vi "A170316-11_Auto.vi"() -> ()   [LabVIEW 2020]
uses:
  Global_Variable/A170316-11.vi
  Global_Variable/Global.vi
  Database/Global1.vi
  <vilib>/addons/database/Connection.llb/DB Tools Open Connec (String).vi
  <vilib>/addons/database/NI_Database_API.lvlib
panel:
  in  "前序OK？":string
  out "拾取检具14":bool
  out "拾取检具13":bool
  out "拾取检具12":bool
  out "拾取检具11":bool
  out "拾取检具10":bool
  out "拾取检具9":bool
  out "拾取检具8":bool
  out "拾取检具7":bool
  out "拾取检具6":bool
  out "拾取检具5":bool
  out "拾取检具4":bool
  out "拾取检具3":bool
  out "拾取检具2":bool
  out "拾取检具1":bool
  out "磨合次数":i32
  in  "STEP":string
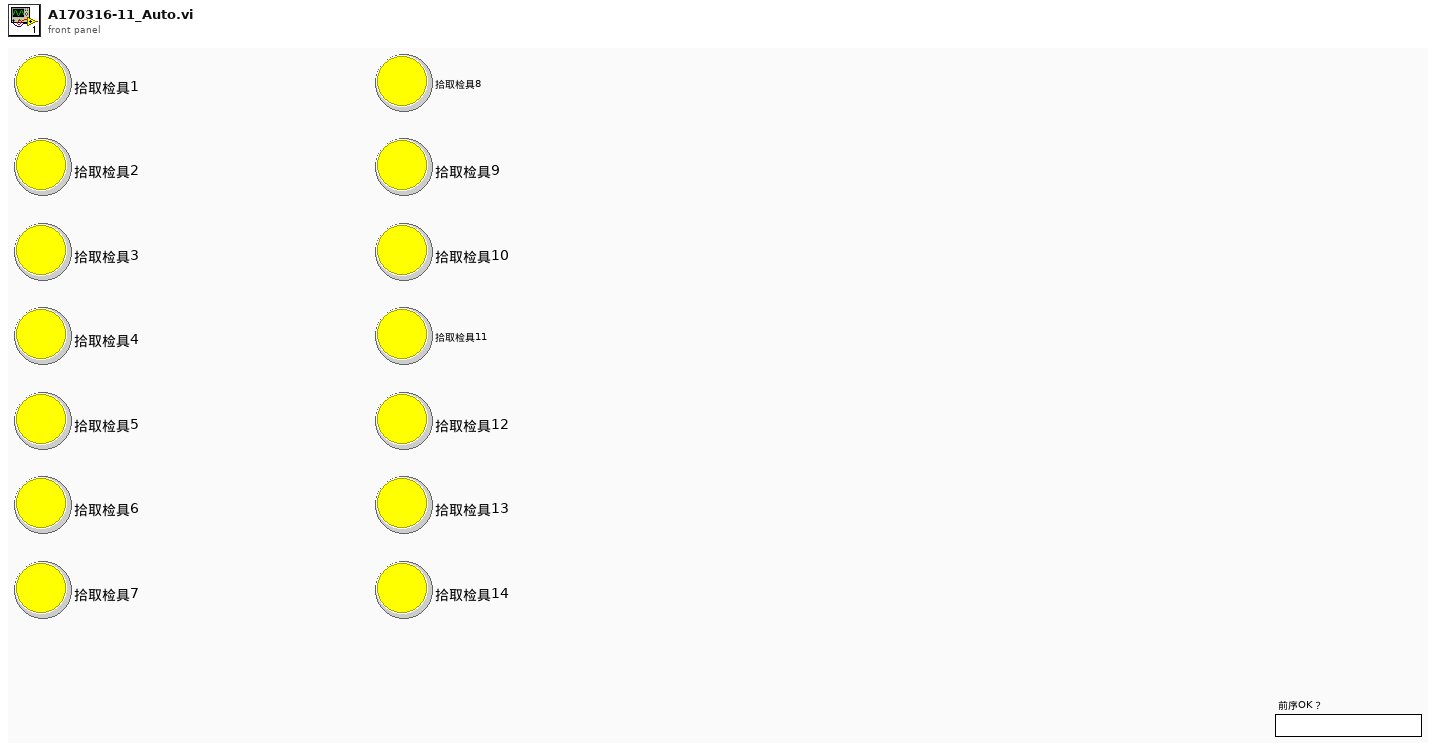
[diagram p1: front panel]
types:
  T1 = enum32{"Invalid", "Standard", "Closed", "Hidden", "Minimized", "Maximized"}
  T2 = cluster{i64, i64, i64, "生产结果":string, "result string":string}
  T3 = cluster{i64, i64, i64, "生产结果":string, "result string":string}[]
  T4 = typedef "NI_Database_API.lvlib/Conn ObjectReference.ctl" = refnum<k1>
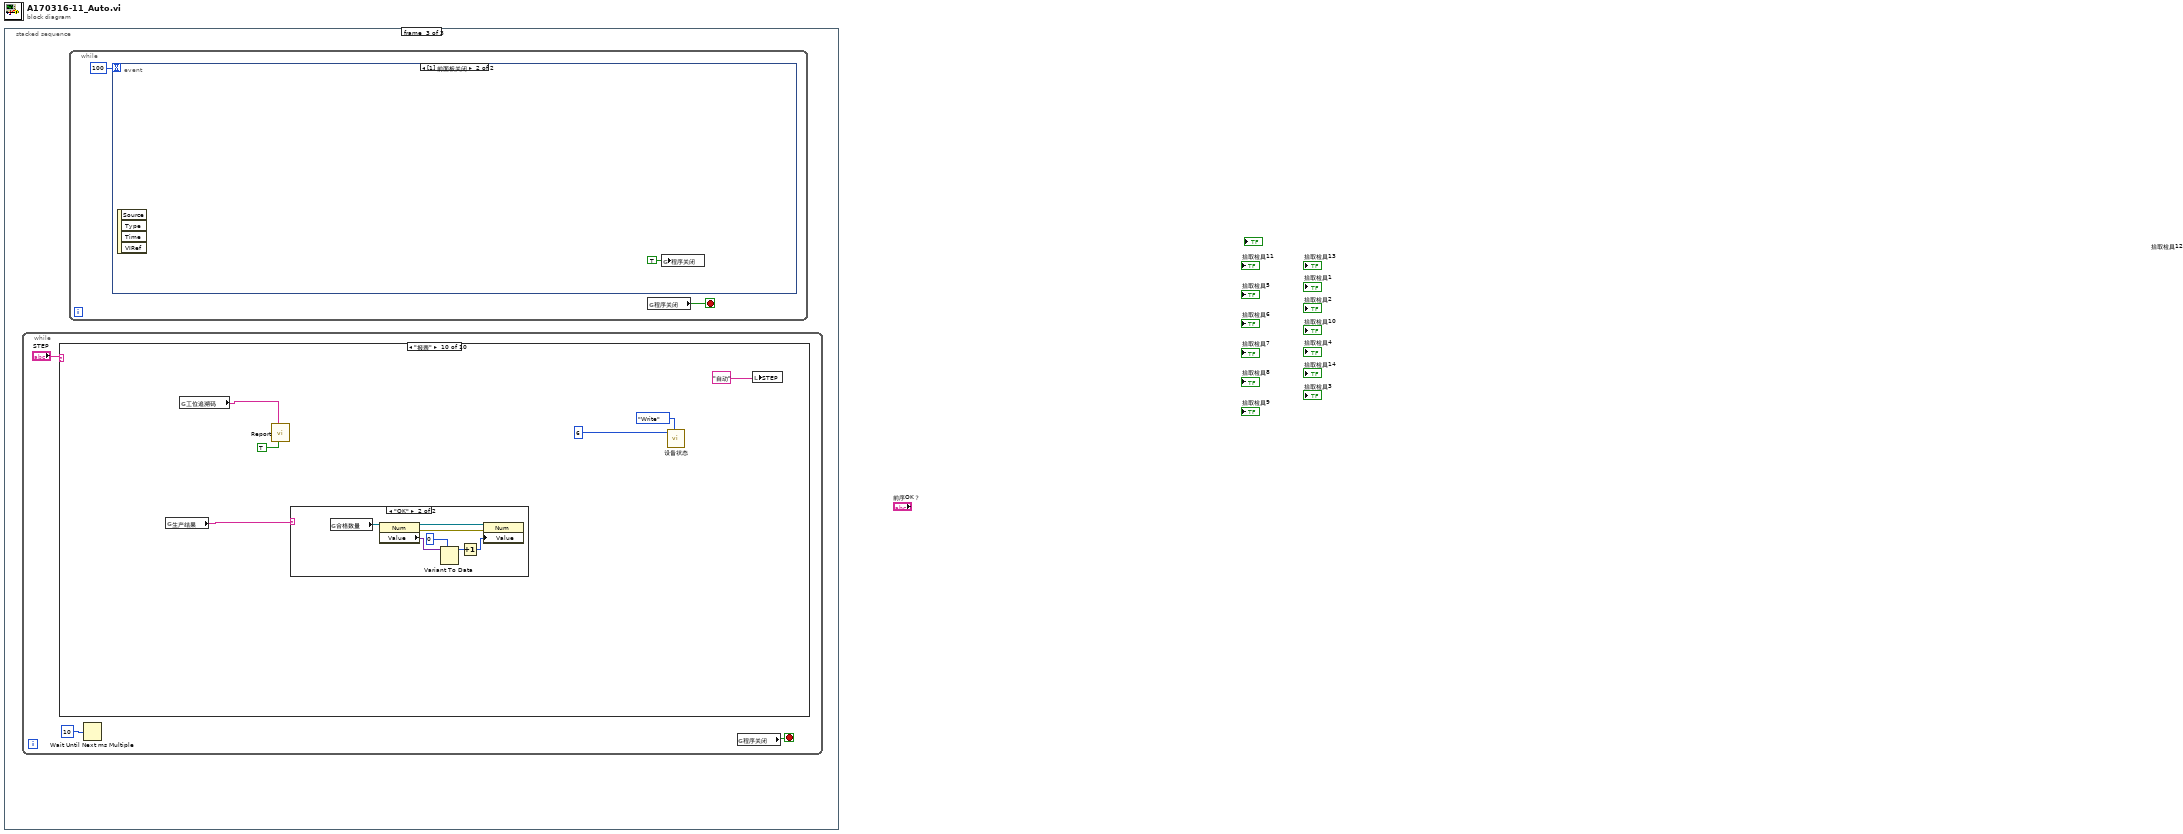
[diagram p0: block diagram]
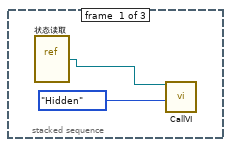
[diagram p2: hidden frame]
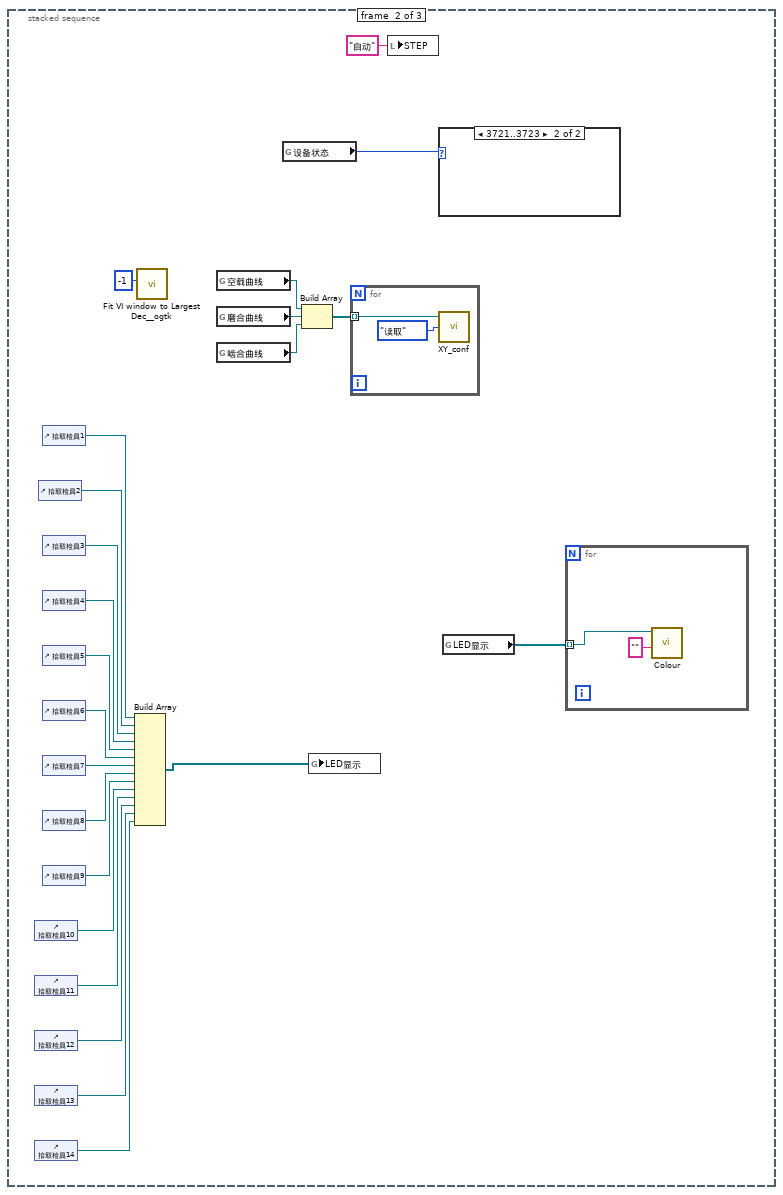
[diagram p3: hidden frame]
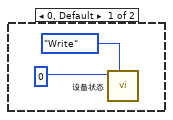
[diagram p4: hidden frame]
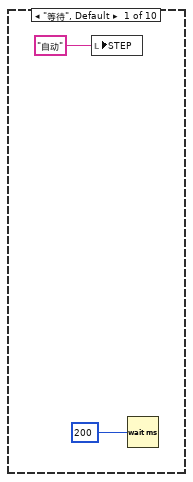
[diagram p5: hidden frame]
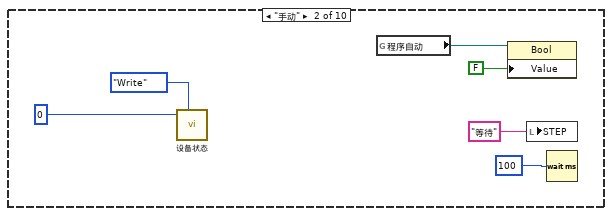
[diagram p6: hidden frame]
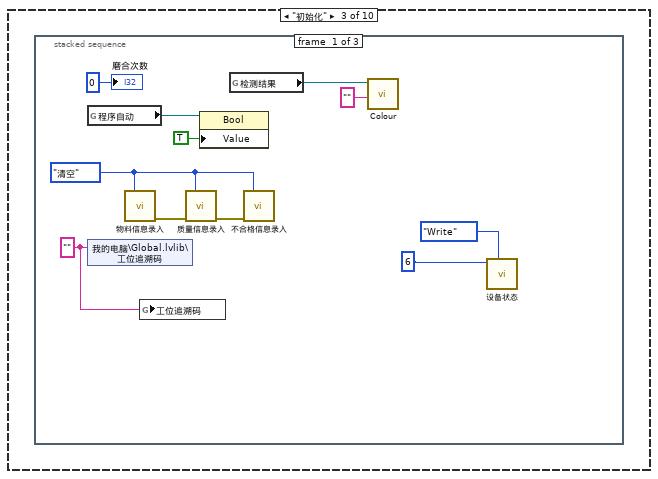
[diagram p7: hidden frame]
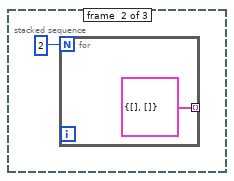
[diagram p8: hidden frame]
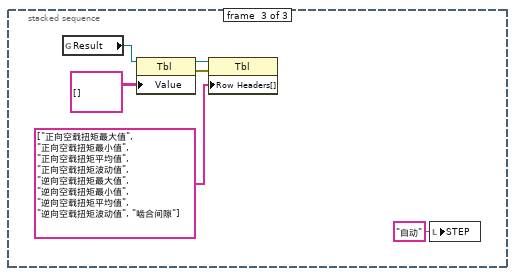
[diagram p9: hidden frame]
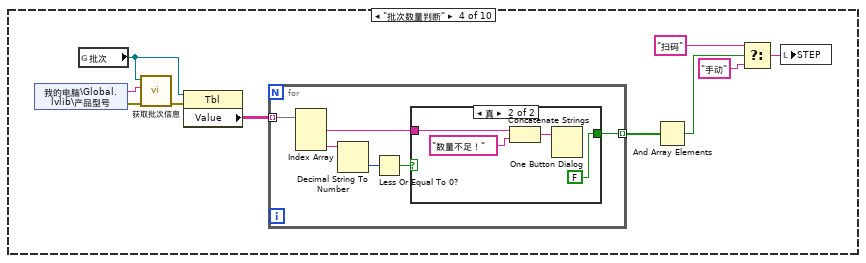
[diagram p10: hidden frame]
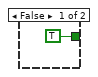
[diagram p11: hidden frame]
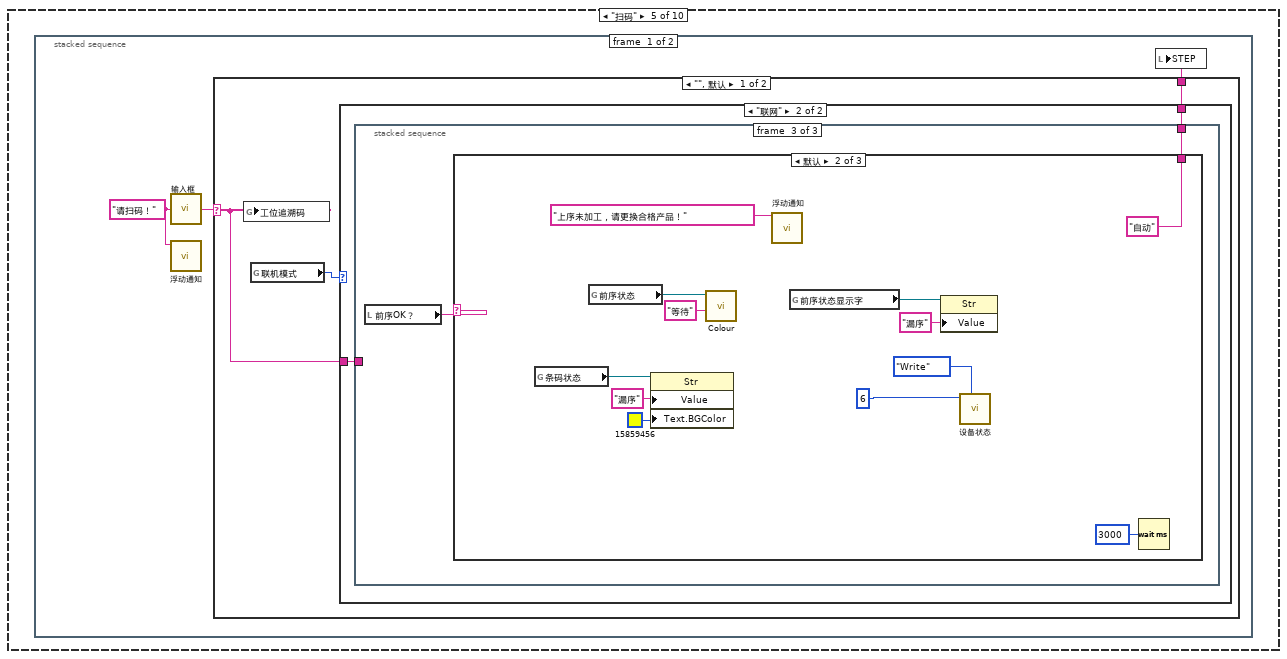
[diagram p12: hidden frame]
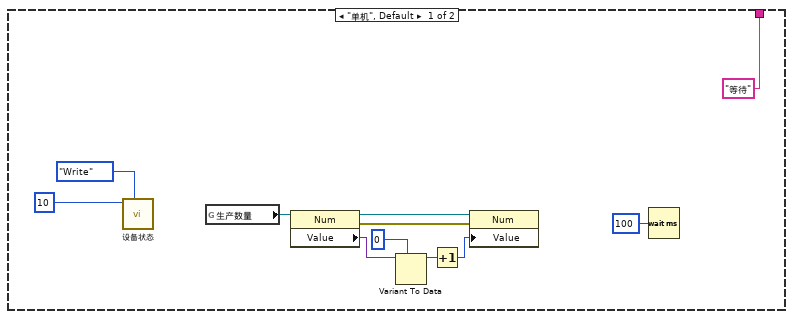
[diagram p13: hidden frame]
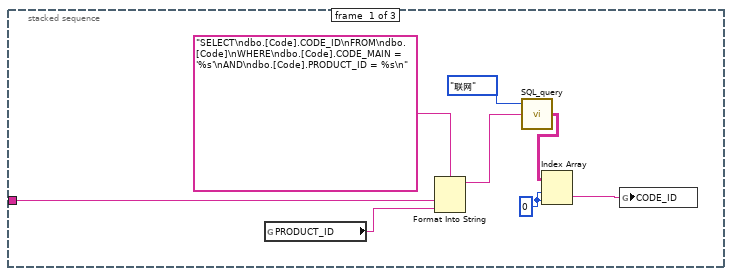
[diagram p14: hidden frame]
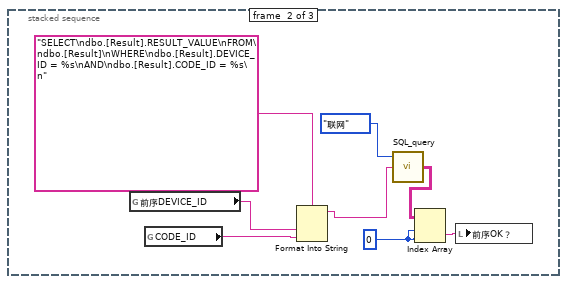
[diagram p15: hidden frame]
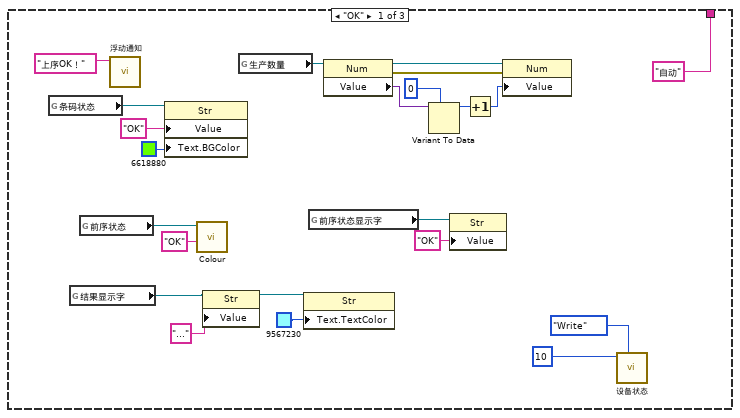
[diagram p16: hidden frame]
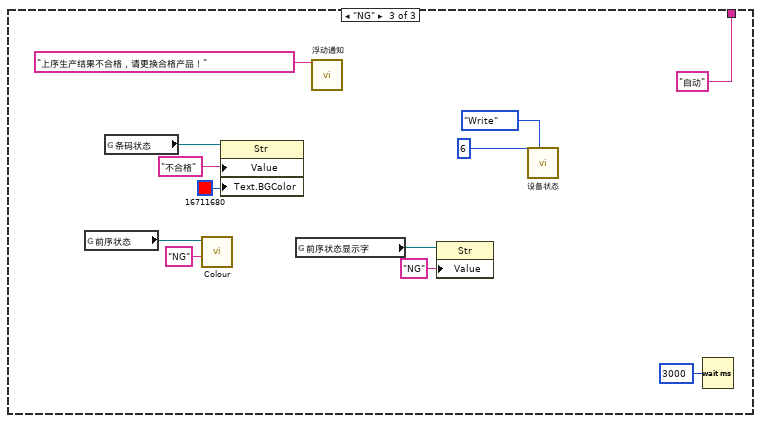
[diagram p17: hidden frame]
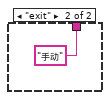
[diagram p18: hidden frame]
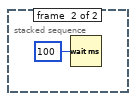
[diagram p19: hidden frame]
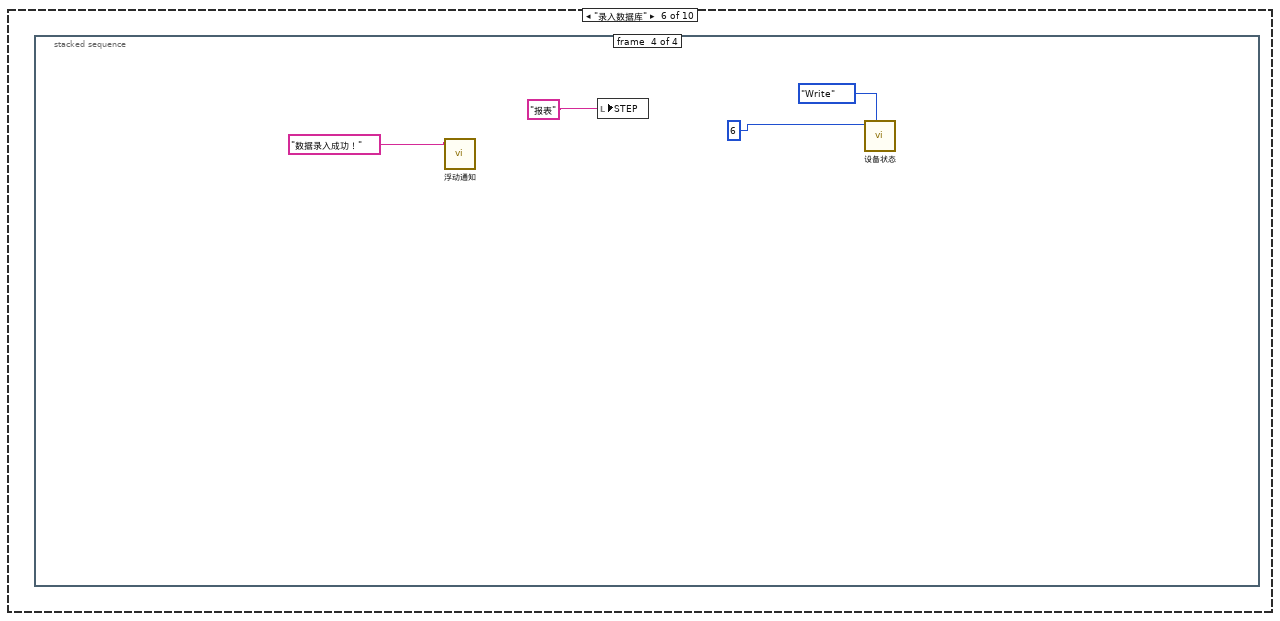
[diagram p20: hidden frame]
diagram:
  n1 = stacked-sequence {
    frame #0 {
      n2 = vi-ref "状态读取.vi"() -> (w1:refnum<vi>)
      n3 = call "CallVI.vi"("VI引用"=w1, "状态"=T1."Hidden") -> ()  [unwired: 11 in, 3 out]
    }
    frame #1 {
      n4 = control-ref of="拾取检具10"() -> (w10:refnum<vi>)
      n5 = control-ref of="拾取检具11"() -> (w9:refnum<vi>)
      n6 = control-ref of="拾取检具12"() -> (w8:refnum<vi>)
      n7 = control-ref of="拾取检具13"() -> (w7:refnum<vi>)
      n8 = control-ref of="拾取检具14"() -> (w6:refnum<vi>)
      n9 = control-ref of="拾取检具2"() -> (w18:refnum<vi>)
      n10 = control-ref of="拾取检具1"() -> (w19:refnum<vi>)
      n11 = control-ref of="拾取检具3"() -> (w17:refnum<vi>)
      n12 = control-ref of="拾取检具4"() -> (w16:refnum<vi>)
      n13 = control-ref of="拾取检具5"() -> (w15:refnum<vi>)
      n14 = control-ref of="拾取检具6"() -> (w14:refnum<vi>)
      n15 = control-ref of="拾取检具7"() -> (w13:refnum<vi>)
      n16 = control-ref of="拾取检具8"() -> (w12:refnum<vi>)
      n17 = control-ref of="拾取检具9"() -> (w11:refnum<vi>)
      n18 = Build Array(w19, w18, w17, w16, w15, w14, w13, w12, w11, w10, w9, w8, w7, w6) -> (w5:refnum<vi>[])
      n19 = call <userlib>:"Fit VI window to Largest Dec__ogtk.vi"("border spacing (2 px)"=-1) -> ()  [unwired: 5 in, 2 out]
      n20 = global read "A170316-11.vi" "空载曲线"() -> (w20:refnum<vi>)
      n21 = global read "A170316-11.vi" "磨合曲线"() -> (w21:refnum<vi>)
      n22 = global read "A170316-11.vi" "啮合曲线"() -> (w22:refnum<vi>)
      n23 = global read "Global.vi" "设备状态"() -> (w3:i32)
      n24 = Build Array(w20, w21, w22) -> (w24:refnum<vi>[])
      n25 = global write "A170316-11.vi" "LED显示"(w5) -> ()
      n26 = for {
        tunnel: w24 -> [w31] mode=indexing
        n27 = call "XY_conf.vi"("方式"=enum16{"写入", "读取"}."读取", "XY图引用"=w31) -> ()  [unwired: 3 in, 1 out]
      }
      n28 = local write "STEP"("自动" ("STEP")) -> ()
      n29 = case shown="3721..3723" w3 {
        frame 0, Default {
          n30 = call "设备状态.vi"("枚举"=enum16{"Read", "Write"}."Write", "Status_Write"=i16 0 ("设备状态")) -> ()  [unwired: 9 in, 1 out]
        }
        frame 3721..3723 {
        }
      }
      n31 = global read "A170316-11.vi" "LED显示"() -> (w4:refnum<vi>[])
      n32 = for {
        tunnel: w4 -> [w27] mode=indexing
        n33 = call "Colour.vi"("result"="", "colourRef"=w27) -> ()  [unwired: 9 in, 1 out]
      }
    }
    frame #2 {
      n34 = while {
        stop <- w33 stop-if-true
        n35 = case shown="\"报表\"" "STEP" {
          frame "等待", Default {
            n36 = local write "STEP"("自动" ("STEP")) -> ()
            n37 = Wait (ms)(milliseconds to wait=u32 200 ("等待时间（毫秒）")) -> ()  [unwired: 1 out]
          }
          frame "手动" {
            n38 = call "设备状态.vi"("枚举"=enum16{"Read", "Write"}."Write", "Status_Write"=u16 0 ("设备状态")) -> ()  [unwired: 9 in, 1 out]
            n39 = global read "Global.vi" "程序自动"() -> (w40:refnum<vi>)
            n40 = property class="Bool"(reference=w40, "Value"=FALSE) -> ()  [unwired: 1 in, 2 out]
            n41 = local write "STEP"("等待" ("STEP")) -> ()
            n42 = Wait (ms)(milliseconds to wait=u32 100 ("等待时间（毫秒）")) -> ()  [unwired: 1 out]
          }
          frame "初始化" {
            n43 = stacked-sequence {
              frame #0 {
                w45 = "" ("传感器码")
                w52 = enum16{"录入", "清空"}."清空" ("功能")
                n44 = global read "Global.vi" "程序自动"() -> (w49:refnum<vi>)
                n45 = shared-variable "我的电脑\\Global.lvlib\\工位追溯码"(w45) -> ()  [unwired: 1 in, 1 out]
                n46 = call "物料信息录入.vi"("功能"=w52) -> ("错误输出"=w51:errorcluster)  [unwired: 14 in]
                n47 = global write "Global1.vi" "工位追溯码"(w45) -> ()
                n48 = call "质量信息录入.vi"("功能"=w52, "错误输入（无错误）"=w51) -> ("错误输出"=w53:errorcluster)  [unwired: 13 in]
                n49 = property class="Bool"(reference=w49, "Value"=TRUE) -> ()  [unwired: 1 in, 2 out]
                n50 = global read "Global.vi" "检测结果"() -> (w47:refnum<vi>)
                n51 = call "不合格信息录入.vi"("功能"=w52, "错误输入（无错误）"=w53) -> ()  [unwired: 13 in, 1 out]
                n52 = call "Colour.vi"("result"="", "colourRef"=w47) -> ()  [unwired: 9 in, 1 out]
                n53 = call "设备状态.vi"("枚举"=enum16{"Read", "Write"}."Write", "Status_Write"=i16 6 ("设备状态")) -> ()  [unwired: 9 in, 1 out]
                "磨合次数" <- 0 ("磨合次数")
              }
              frame #1 {
                n54 = for {
                  N: 2 -> [_]
                  tunnel: [cluster{dbl[], dbl[]} {[], []}] -> _ mode=indexing
                }
              }
              frame #2 {
                n55 = global read "Global.vi" "Result"() -> (w59:refnum<vi>)
                n56 = property class="Tbl"(reference=w59, "Value"=string[][] []) -> (reference out=w60:refnum<vi>, error out=w61:errorcluster)  [unwired: 1 in]
                n57 = property class="Tbl"(reference=w60, error in=w61, "Row Headers[]"=string[] ["正向空载扭矩最大值", "正向空载扭矩最小值", "正向空载扭矩平均值", "正向空载扭矩波动值", "逆向空载扭矩最大值", "逆向空载扭矩最小值", "逆向空载扭矩平均值", "逆向空载扭矩波动值", "啮合间隙"] ("列首字符串[]")) -> ()  [unwired: 2 out]
                n58 = local write "STEP"("自动" ("STEP")) -> ()
              }
            }
          }
          frame "批次数量判断" {
            n59 = shared-variable "我的电脑\\Global.lvlib\\产品型号"() -> (w67:string, error out=w70:errorcluster)  [unwired: 1 in]
            n60 = global read "Global.vi" "批次"() -> (w68:refnum<vi>)
            n61 = call "获取批次信息.vi"("error in (no error)"=w70, "产品型号"=w67, "Tbl引用句柄"=w68) -> ("error out"=w69:errorcluster)  [unwired: 7 in, 1 out]
            n62 = property class="Tbl"(reference=w68, error in=w69) -> ("Value"=w71:string[][])  [unwired: 2 out]
            n63 = for {
              tunnel: w71 -> [w77] mode=indexing
              tunnel: [w72] -> w66 mode=indexing
              n64 = Index Array(array=w77) -> (element #1=w73:string, element #3=w76:string)  [unwired: 3 in, 1 out]
              n65 = Decimal String To Number(string=w76) -> (number=w75:i32)  [unwired: 2 in, 1 out]
              n66 = Less Or Equal To 0?(x=w75) -> (x <= 0?=w74:bool)
              n67 = case shown="真" w74 {
                tunnel: w73 -> [_ w82]
                tunnel: [TRUE FALSE] -> w72
                frame False {
                }
                frame True {
                  n68 = Concatenate Strings(w82, "数量不足！" ("字符串")) -> (w80:string)
                  n69 = One Button Dialog(message=w80) -> ()  [unwired: 1 in, 1 out]
                }
              }
            }
            n70 = And Array Elements(Boolean array=w66) -> (logical AND=w65:bool)
            n71 = Select(t="扫码" ("STEP"), s=w65, f="手动" ("STEP")) -> (s? t:f=w62:string)
            n72 = local write "STEP"(w62) -> ()
          }
          frame "扫码" {
            n73 = stacked-sequence {
              frame #0 {
                w84 = "请扫码！" ("提示信息")
                n74 = call "输入框.vi"("提示信息"=w84) -> ("条形码输出"=w85:string)
                n75 = call "浮动通知.vi"("通知内容"=w84) -> ()  [unwired: 11 in]
                n76 = case shown="\"\", 默认" w85 {
                  selector: w85 -> [w86 _]
                  tunnel: [w87 "手动"] -> w83
                  frame "", Default {
                    n77 = global write "Global1.vi" "工位追溯码"(w86) -> ()
                    n78 = global read "Global1.vi" "联机模式"() -> (w88:enum16{"单机", "联网"})
                    n79 = case shown="\"联网\"" w88 {
                      tunnel: ["等待" ("State(s) in Front (\"\")") w100] -> w87
                      tunnel: w86 -> [_ w101]
                      frame "单机", Default {
                        n80 = call "设备状态.vi"("枚举"=enum16{"Read", "Write"}."Write", "Status_Write"=i16 10 ("设备状态控制字")) -> ()  [unwired: 9 in, 1 out]
                        n81 = global read "Global.vi" "生产数量"() -> (w97:refnum<vi>)
                        n82 = property class="Num"(reference=w97) -> (reference out=w96:refnum<vi>, error out=w95:errorcluster, "Value"=w94:variant)  [unwired: 1 in]
                        n83 = Variant To Data(type=u32 0, Variant=w94) -> (data=w93:u32)  [unwired: 1 in, 1 out]
                        n84 = Increment(x=w93) -> (x+1=w92:u32)
                        n85 = property class="Num"(reference=w96, error in=w95, "Value"=w92) -> ()  [unwired: 2 out]
                        n86 = Wait (ms)(milliseconds to wait=u32 100 ("等待时间（毫秒）")) -> ()  [unwired: 1 out]
                      }
                      frame "联网" {
                        n87 = stacked-sequence {
                          tunnel: w101 -> [w107 _ _]
                          tunnel: [_ _ w118] -> w100
                          frame #0 {
                            w102 = 0 ("索引 (行)")
                            n88 = global read "Global1.vi" "PRODUCT_ID"() -> (w108:string)
                            n89 = Format Into String(format string="SELECT\ndbo.[Code].CODE_ID\nFROM\ndbo.[Code]\nWHERE\ndbo.[Code].CODE_MAIN = '%s'\nAND\ndbo.[Code].PRODUCT_ID = %s\n" ("格式字符串"), w107, w108) -> (resulting string=w106:string)  [unwired: 2 in, 1 out]
                            n90 = call "SQL_query.vi"("SQL query"=w106, "联机模式"=enum16{"单机", "联网"}."联网") -> ("data"=w104:string[][])  [unwired: 1 in, 2 out]
                            n91 = Index Array(array=w104, index (row)=w102, index (col)=w102) -> (element=w103:string)
                            n92 = global write "Global1.vi" "CODE_ID"(w103) -> ()
                          }
                          frame #1 {
                            w110 = 0 ("索引 (行)")
                            n93 = global read "Global1.vi" "前序DEVICE_ID"() -> (w116:string)
                            n94 = global read "Global1.vi" "CODE_ID"() -> (w117:string)
                            n95 = Format Into String(format string="SELECT\ndbo.[Result].RESULT_VALUE\nFROM\ndbo.[Result]\nWHERE\ndbo.[Result].DEVICE_ID = %s\nAND\ndbo.[Result].CODE_ID = %s\n" ("格式字符串"), w116, w117) -> (resulting string=w113:string)  [unwired: 2 in, 1 out]
                            n96 = call "SQL_query.vi"("SQL query"=w113, "联机模式"=enum16{"单机", "联网"}."联网") -> ("data"=w112:string[][])  [unwired: 1 in, 2 out]
                            n97 = Index Array(array=w112, index (row)=w110, index (col)=w110) -> (element=w111:string)
                            n98 = local write "前序OK？"(w111) -> ()
                          }
                          frame #2 {
                            n99 = local read "前序OK？"() -> (w119:string)
                            n100 = case shown="默认" w119 {
                              tunnel: ["自动" "自动" "自动"] -> w118
                              frame "OK" {
                                n101 = global read "Global.vi" "条码状态"() -> (w122:refnum<vi>)
                                n102 = global read "Global.vi" "结果显示字"() -> (w127:refnum<vi>)
                                n103 = global read "Global.vi" "前序状态"() -> (w132:refnum<vi>)
                                n104 = call "浮动通知.vi"("通知内容"="上序OK！" ("Status")) -> ()  [unwired: 11 in]
                                n105 = property class="Str"(reference=w122, "Value"="OK" ("result"), "Text.BGColor"=u32 6618880 ("文本.文本颜色:背景色")) -> ()  [unwired: 1 in, 2 out]
                                n106 = call "Colour.vi"("result"="OK", "colourRef"=w132) -> ()  [unwired: 9 in, 1 out]
                                n107 = property class="Str"(reference=w127, "Value"="..." ("值")) -> (reference out=w126:refnum<vi>)  [unwired: 1 in, 1 out]
                                n108 = global read "Global.vi" "生产数量"() -> (w138:refnum<vi>)
                                n109 = property class="Str"(reference=w126, "Text.TextColor"=u32 9567230) -> ()  [unwired: 1 in, 2 out]
                                n110 = global read "Global.vi" "前序状态显示字"() -> (w130:refnum<vi>)
                                n111 = property class="Num"(reference=w138) -> (reference out=w137:refnum<vi>, error out=w136:errorcluster, "Value"=w135:variant)  [unwired: 1 in]
                                n112 = Variant To Data(type=u32 0, Variant=w135) -> (data=w134:u32)  [unwired: 1 in, 1 out]
                                n113 = property class="Str"(reference=w130, "Value"="OK" ("值")) -> ()  [unwired: 1 in, 2 out]
                                n114 = Increment(x=w134) -> (x+1=w133:u32)
                                n115 = property class="Num"(reference=w137, error in=w136, "Value"=w133) -> ()  [unwired: 2 out]
                                n116 = call "设备状态.vi"("枚举"=enum16{"Read", "Write"}."Write", "Status_Write"=i16 10 ("设备状态控制字")) -> ()  [unwired: 9 in, 1 out]
                              }
                              frame Default {
                                n117 = global read "Global.vi" "条码状态"() -> (w144:refnum<vi>)
                                n118 = global read "Global.vi" "前序状态"() -> (w150:refnum<vi>)
                                n119 = property class="Str"(reference=w144, "Value"="漏序" ("result"), "Text.BGColor"=u32 15859456 ("文本.文本颜色:背景色")) -> ()  [unwired: 1 in, 2 out]
                                n120 = call "Colour.vi"("result"="等待", "colourRef"=w150) -> ()  [unwired: 9 in, 1 out]
                                n121 = call "浮动通知.vi"("通知内容"="上序未加工，请更换合格产品！" ("Status")) -> ()  [unwired: 11 in]
                                n122 = global read "Global.vi" "前序状态显示字"() -> (w148:refnum<vi>)
                                n123 = property class="Str"(reference=w148, "Value"="漏序" ("值")) -> ()  [unwired: 1 in, 2 out]
                                n124 = call "设备状态.vi"("枚举"=enum16{"Read", "Write"}."Write", "Status_Write"=i16 6 ("设备状态控制字")) -> ()  [unwired: 9 in, 1 out]
                                n125 = Wait (ms)(milliseconds to wait=u32 3000 ("等待时间（毫秒）")) -> ()  [unwired: 1 out]
                              }
                              frame "NG" {
                                n126 = global read "Global.vi" "前序状态"() -> (w162:refnum<vi>)
                                n127 = global read "Global.vi" "条码状态"() -> (w156:refnum<vi>)
                                n128 = call "Colour.vi"("result"="NG", "colourRef"=w162) -> ()  [unwired: 9 in, 1 out]
                                n129 = property class="Str"(reference=w156, "Value"="不合格" ("result"), "Text.BGColor"=u32 16711680 ("文本.文本颜色:背景色")) -> ()  [unwired: 1 in, 2 out]
                                n130 = global read "Global.vi" "前序状态显示字"() -> (w160:refnum<vi>)
                                n131 = call "浮动通知.vi"("通知内容"="上序生产结果不合格，请更换合格产品！" ("Status")) -> ()  [unwired: 11 in]
                                n132 = property class="Str"(reference=w160, "Value"="NG" ("值")) -> ()  [unwired: 1 in, 2 out]
                                n133 = call "设备状态.vi"("枚举"=enum16{"Read", "Write"}."Write", "Status_Write"=i16 6 ("设备状态控制字")) -> ()  [unwired: 9 in, 1 out]
                                n134 = Wait (ms)(milliseconds to wait=u32 3000 ("等待时间（毫秒）")) -> ()  [unwired: 1 out]
                              }
                            }
                          }
                        }
                      }
                    }
                  }
                  frame "exit" {
                  }
                }
                n135 = local write "STEP"(w83) -> ()
              }
              frame #1 {
                n136 = Wait (ms)(milliseconds to wait=u32 100 ("等待时间（毫秒）")) -> ()  [unwired: 1 out]
              }
            }
          }
          frame "录入数据库" {
            n137 = stacked-sequence {
              frame #0 {
                n138 = Get Date/Time String(date format (0)=enum16{"short", "long", "abbreviated"}."short" ("日期格式(0)"), want seconds? (F)=FALSE ("需要秒？(F)")) -> (date string=w177:string, time string=w178:string)  [unwired: 1 in]
                n139 = global read "Global1.vi" "DEVICE_ID"() -> (w181:string)
                n140 = global read "Global1.vi" "USER_ID"() -> (w179:string)
                n141 = global read "Global1.vi" "CODE_ID"() -> (w180:string)
                n142 = global read "Global1.vi" "生产结果"() -> (w172:string)
                n143 = Concatenate Strings(w177, " " ("字符串"), w178) -> (w173:string)
                n144 = Decimal String To Number(string=w181, default (0L)=i64 0 ("默认(0 I32)")) -> (number=w170:i64)  [unwired: 1 in, 1 out]
                n145 = Decimal String To Number(string=w179, default (0L)=i64 0 ("默认(0 I32)")) -> (number=w169:i64)  [unwired: 1 in, 1 out]
                n146 = Decimal String To Number(string=w180, default (0L)=i64 0 ("默认(0 I32)")) -> (number=w168:i64)  [unwired: 1 in, 1 out]
                n147 = global read "Global1.vi" "联机模式"() -> (w188:enum16{"单机", "联网"})
                n148 = Search and Replace String(replace all?=TRUE ("替换全部？(F)"), input string=w173, search string="/" ("替换字符串(\"\")"), replace string="-" ("替换字符串(\"\")")) -> (result string=w171:string)  [unwired: 4 in, 3 out]
                n149 = Bundle(w170, w169, w168, "生产结果"=w172, "result string"=w171) -> (w194:T2)  [unwired: 1 in]
                n150 = call "GetSQLstring.vi"("联机模式"=w188) -> ("错误输出"=w191:errorcluster, "连接字符串"=w190:string)  [unwired: 9 in]
                n151 = Build Array(w194) -> (w195:T3)
                n152 = call-poly <vilib>:"DB Tools Open Connection.vi"("error in (no error)"=w191, "connection information"=w190) -> ("error out"=w189:errorcluster, "connection reference"=w192:T4)  [unwired: 6 in]
                n153 = for {
                  tunnel: w195 -> [w200] mode=indexing
                  tunnel: w192 -> [w198]
                  shift-right: [w196] -> w193
                  shift-left: w189 -> [w203]
                  w199 = string[] ["DEVICE_ID", "USER_ID", "CODE_ID", "RESULT_VALUE", "RESULT_TIME"] ("columns")
                  w201 = "Result" ("table")
                  n154 = call <vilib>:"DB Tools Insert Data.vi"("data"=w200, "error in (no error)"=w203, "columns"=w199, "table"=w201, "connection reference"=w198) -> ("error out"=w202:errorcluster, "connection reference out"=w197:T4)  [unwired: 5 in]
                  n155 = case shown="错误" w202 {
                    selector: w202 -> [w204 w225]
                    tunnel: w199 -> [_ w222]
                    tunnel: w197 -> [w205 w214]
                    tunnel: w201 -> [_ w226]
                    tunnel: w200 -> [_ w218]
                    tunnel: [w205 w213] -> _
                    tunnel: [w204 w212] -> w196
                    frame No Error {
                    }
                    frame Error {
                      n156 = Array Subset(array=w222, index=3 ("长度"), length=2 ("长度")) -> (w223:string[])
                      n157 = Unbundle(w218) -> (w207:i64, w210:i64, "生产结果"=w217:string, "result string"=w216:string)  [unwired: 1 out]
                      n158 = Number To Decimal String(number=w210) -> (decimal integer string=w211:string)  [unwired: 1 in]
                      n159 = Number To Decimal String(number=w207) -> (decimal integer string=w206:string)  [unwired: 1 in]
                      n160 = Concatenate Strings("WHERE CODE_ID =" ("condition"), w211, "AND DEVICE_ID = ", w206) -> (w219:string)
                      n161 = Bundle("生产结果"=w217, "result string"=w216) -> (w215:cluster{"生产结果":string, "result string":string})  [unwired: 1 in]
                      n162 = call <vilib>:"Clear Errors.vi"("error in (no error)"=w225) -> ("error out"=w224:errorcluster)  [unwired: 5 in, 1 out]
                      n163 = call <vilib>:"DB Tools Update Data.vi"("condition"=w219, "data"=w215, "error in (no error)"=w224, "columns"=w223, "table"=w226, "connection reference"=w214) -> ("error out"=w212:errorcluster, "connection reference out"=w213:T4)  [unwired: 4 in]
                    }
                  }
                }
                n164 = call <vilib>:"Simple Error Handler.vi"("error in (no error)"=w193) -> ()  [unwired: 4 in, 5 out]
              }
              frame #1 {
                n165 = disable-structure shown="禁用" {
                  frame Disabled {
                    n166 = global read "Global1.vi" "控制器码"() -> (w229:string)
                    n167 = global read "Global1.vi" "CODE_ID"() -> (w230:string)
                    n168 = Format Into String(format string="UPDATE\ndbo.[Code]\nSET dbo.[Code].CODE_ECU = '%s'\n\nWHERE\ndbo.[Code].CODE_ID = %s\n" ("格式字符串"), w229, w230) -> (resulting string=w227:string)  [unwired: 2 in, 1 out]
                    n169 = call "SQL_query.vi"("SQL query"=w227, "联机模式"=enum16{"单机", "联网"}."联网") -> ()  [unwired: 1 in, 3 out]
                  }
                  frame Enabled {
                  }
                }
              }
              frame #2 {
              }
              frame #3 {
                n170 = call "浮动通知.vi"("通知内容"="数据录入成功！" ("Status")) -> ()  [unwired: 11 in]
                n171 = local write "STEP"("报表" ("STEP")) -> ()
                n172 = call "设备状态.vi"("枚举"=enum16{"Read", "Write"}."Write", "Status_Write"=i16 6 ("设备状态")) -> ()  [unwired: 9 in, 1 out]
              }
            }
          }
          frame "录入批次" {
            n173 = shared-variable "我的电脑\\Global.lvlib\\产品型号"() -> (w237:string)  [unwired: 1 in, 1 out]
            n174 = call "更新批次.vi"("型号"=w237) -> ("error out"=w238:errorcluster)  [unwired: 10 in]
            n175 = global read "Global.vi" "批次"() -> (w239:refnum<vi>)
            n176 = call "更新易损件.vi"("error in (no error)"=w238) -> ("error out"=w241:errorcluster)  [unwired: 10 in]
            n177 = property class="Tbl"(reference=w239, error in=w241) -> ("Value"=w240:string[][])  [unwired: 2 out]
            n178 = for {
              tunnel: w240 -> [w244] mode=indexing
              n179 = Index Array(array=w244) -> (element #1=w243:string, element #2=w242:string)  [unwired: 2 in]
              n180 = call "物料信息录入.vi"("物料名称"=w243, "功能"=enum16{"录入", "清空"}."录入", "物料编码"=w242) -> ()  [unwired: 12 in, 1 out]
            }
            n181 = local write "STEP"("等待" ("STEP")) -> ()
          }
          frame "自动" {
            n182 = global read "Global.vi" "设备状态"() -> (w246:i32)
            n183 = global read "A170316-11.vi" "LED显示"() -> (w247:refnum<vi>[])
            n184 = case shown="202" w246 {
              tunnel: w247 -> [_ _ _ _ w256 _ _ w264 _ w274 _ w286 _ w298 _ w310 _ w322 _ w334 _ w346 _ w357 _ w368 _ w380 _ w392 _ w404 _ w416 _ w428 _ w439 _ _ _ _ _ _]
              frame Default {
              }
              frame -128 {
                n185 = call "浮动通知.vi"("通知内容"="复位中……" ("Status")) -> ()  [unwired: 11 in]
                n186 = global read "Global.vi" "程序自动"() -> (w249:refnum<vi>)
                n187 = property class="Bool"(reference=w249, "Value"=FALSE) -> ()  [unwired: 1 in, 2 out]
              }
              frame 5 {
                n188 = call "浮动通知.vi"("通知内容"="复位完成" ("Status")) -> ()  [unwired: 11 in]
              }
              frame 0 {
                n189 = call "浮动通知.vi"("通知内容"="不在自动！" ("Status")) -> ()  [unwired: 11 in]
              }
              frame 6 {
                n190 = for {
                  tunnel: w256 -> [w258] mode=indexing
                  n191 = call "Colour.vi"("result"="", "colourRef"=w258) -> ()  [unwired: 9 in, 1 out]
                }
                n192 = global write "Global1.vi" "工位追溯码"("" ("工位追溯码")) -> ()
                n193 = Wait (ms)(milliseconds to wait=u32 1000 ("等待时间（毫秒）")) -> ()  [unwired: 1 out]
                n194 = call "浮动通知.vi"("通知内容"="请扫码！" ("Status")) -> ()  [unwired: 11 in]
                n195 = local write "STEP"("扫码" ("STEP")) -> ()
              }
              frame 8 {
                n196 = call "浮动通知.vi"("通知内容"="程序停止！" ("Status")) -> ()  [unwired: 11 in]
              }
              frame 9 {
                n197 = call "浮动通知.vi"("通知内容"="套花键中" ("Status")) -> ()  [unwired: 11 in]
              }
              frame 10 {
                n198 = Index Array(array=w264, index=0 ("索引")) -> (element=w266:refnum<vi>)
                n199 = call "Colour.vi"("result"="等待", "colourRef"=w266) -> ()  [unwired: 9 in, 1 out]
                n200 = call "浮动通知.vi"("通知内容"="请拾取检具1！" ("Status")) -> ()  [unwired: 11 in]
                n201 = call "设备状态.vi"("枚举"=enum16{"Read", "Write"}."Write", "Status_Write"=i16 11 ("设备状态")) -> ()  [unwired: 9 in, 1 out]
              }
              frame 12 {
                n202 = call "浮动通知.vi"("通知内容"="请放回检具1！" ("Status")) -> ()  [unwired: 11 in]
                n203 = call "设备状态.vi"("枚举"=enum16{"Read", "Write"}."Write", "Status_Write"=i16 13 ("设备状态")) -> ()  [unwired: 9 in, 1 out]
              }
              frame 14 {
                n204 = Index Array(array=w274, index #1=0 ("索引")) -> (element #1=w280:refnum<vi>, element #2=w279:refnum<vi>)  [unwired: 1 in]
                n205 = call "浮动通知.vi"("通知内容"="请拾取检具2！" ("Status")) -> ()  [unwired: 11 in]
                n206 = call "设备状态.vi"("枚举"=enum16{"Read", "Write"}."Write", "Status_Write"=i16 20 ("设备状态")) -> ()  [unwired: 9 in, 1 out]
                n207 = call "Colour.vi"("result"="OK", "colourRef"=w280) -> ()  [unwired: 9 in, 1 out]
                n208 = call "Colour.vi"("result"="等待", "colourRef"=w279) -> ()  [unwired: 9 in, 1 out]
              }
              frame 21 {
                n209 = call "浮动通知.vi"("通知内容"="请放回检具2！" ("Status")) -> ()  [unwired: 11 in]
                n210 = call "设备状态.vi"("枚举"=enum16{"Read", "Write"}."Write", "Status_Write"=i16 23 ("设备状态")) -> ()  [unwired: 9 in, 1 out]
              }
              frame 25 {
                n211 = Index Array(array=w286, index #1=1 ("索引")) -> (element #1=w291:refnum<vi>, element #2=w287:refnum<vi>)  [unwired: 1 in]
                n212 = call "浮动通知.vi"("通知内容"="请拾取检具3！" ("Status")) -> ()  [unwired: 11 in]
                n213 = call "Colour.vi"("result"="等待", "colourRef"=w287) -> ()  [unwired: 9 in, 1 out]
                n214 = call "Colour.vi"("result"="OK", "colourRef"=w291) -> ()  [unwired: 9 in, 1 out]
                n215 = call "设备状态.vi"("枚举"=enum16{"Read", "Write"}."Write", "Status_Write"=i16 30 ("设备状态")) -> ()  [unwired: 9 in, 1 out]
              }
              frame 31 {
                n216 = call "浮动通知.vi"("通知内容"="请放回检具3！" ("Status")) -> ()  [unwired: 11 in]
                n217 = call "设备状态.vi"("枚举"=enum16{"Read", "Write"}."Write", "Status_Write"=i16 33 ("设备状态")) -> ()  [unwired: 9 in, 1 out]
              }
              frame 35 {
                n218 = Index Array(array=w298, index #1=2 ("索引")) -> (element #1=w303:refnum<vi>, element #2=w299:refnum<vi>)  [unwired: 1 in]
                n219 = call "浮动通知.vi"("通知内容"="请拾取检具4！" ("Status")) -> ()  [unwired: 11 in]
                n220 = call "Colour.vi"("result"="OK", "colourRef"=w303) -> ()  [unwired: 9 in, 1 out]
                n221 = call "Colour.vi"("result"="等待", "colourRef"=w299) -> ()  [unwired: 9 in, 1 out]
                n222 = call "设备状态.vi"("枚举"=enum16{"Read", "Write"}."Write", "Status_Write"=i16 40 ("设备状态")) -> ()  [unwired: 9 in, 1 out]
              }
              frame 41 {
                n223 = call "浮动通知.vi"("通知内容"="请放回检具4！" ("Status")) -> ()  [unwired: 11 in]
                n224 = call "设备状态.vi"("枚举"=enum16{"Read", "Write"}."Write", "Status_Write"=i16 43 ("设备状态")) -> ()  [unwired: 9 in, 1 out]
              }
              frame 45 {
                n225 = Index Array(array=w310, index #1=3 ("索引")) -> (element #1=w315:refnum<vi>, element #2=w311:refnum<vi>)  [unwired: 1 in]
                n226 = call "浮动通知.vi"("通知内容"="请拾取检具5！" ("Status")) -> ()  [unwired: 11 in]
                n227 = call "Colour.vi"("result"="OK", "colourRef"=w315) -> ()  [unwired: 9 in, 1 out]
                n228 = call "Colour.vi"("result"="等待", "colourRef"=w311) -> ()  [unwired: 9 in, 1 out]
                n229 = call "设备状态.vi"("枚举"=enum16{"Read", "Write"}."Write", "Status_Write"=i16 50 ("设备状态")) -> ()  [unwired: 9 in, 1 out]
              }
              frame 51 {
                n230 = call "浮动通知.vi"("通知内容"="请放回检具5！" ("Status")) -> ()  [unwired: 11 in]
                n231 = call "设备状态.vi"("枚举"=enum16{"Read", "Write"}."Write", "Status_Write"=i16 53 ("设备状态")) -> ()  [unwired: 9 in, 1 out]
              }
              frame 55 {
                n232 = Index Array(array=w322, index #1=4 ("索引")) -> (element #1=w326:refnum<vi>, element #2=w323:refnum<vi>)  [unwired: 1 in]
                n233 = call "浮动通知.vi"("通知内容"="请拾取检具6！" ("Status")) -> ()  [unwired: 11 in]
                n234 = call "Colour.vi"("result"="OK", "colourRef"=w326) -> ()  [unwired: 9 in, 1 out]
                n235 = call "Colour.vi"("result"="等待", "colourRef"=w323) -> ()  [unwired: 9 in, 1 out]
                n236 = call "设备状态.vi"("枚举"=enum16{"Read", "Write"}."Write", "Status_Write"=i16 60 ("设备状态")) -> ()  [unwired: 9 in, 1 out]
              }
              frame 61 {
                n237 = call "浮动通知.vi"("通知内容"="请放回检具6！" ("Status")) -> ()  [unwired: 11 in]
                n238 = call "设备状态.vi"("枚举"=enum16{"Read", "Write"}."Write", "Status_Write"=i16 63 ("设备状态")) -> ()  [unwired: 9 in, 1 out]
              }
              frame 65 {
                n239 = Index Array(array=w334, index #1=5 ("索引")) -> (element #1=w339:refnum<vi>, element #2=w335:refnum<vi>)  [unwired: 1 in]
                n240 = call "浮动通知.vi"("通知内容"="请拾取检具7！" ("Status")) -> ()  [unwired: 11 in]
                n241 = call "设备状态.vi"("枚举"=enum16{"Read", "Write"}."Write", "Status_Write"=i16 70 ("设备状态")) -> ()  [unwired: 9 in, 1 out]
                n242 = call "Colour.vi"("result"="等待", "colourRef"=w335) -> ()  [unwired: 9 in, 1 out]
                n243 = call "Colour.vi"("result"="OK", "colourRef"=w339) -> ()  [unwired: 9 in, 1 out]
              }
              frame 71 {
                n244 = call "浮动通知.vi"("通知内容"="请放回检具7！" ("Status")) -> ()  [unwired: 11 in]
                n245 = call "设备状态.vi"("枚举"=enum16{"Read", "Write"}."Write", "Status_Write"=i16 73 ("设备状态")) -> ()  [unwired: 9 in, 1 out]
              }
              frame 75 {
                n246 = Index Array(array=w346, index=6 ("索引")) -> (element=w350:refnum<vi>)
                n247 = call "浮动通知.vi"("通知内容"="请拾取检具8！" ("Status")) -> ()  [unwired: 11 in]
                n248 = call "Colour.vi"("result"="等待") -> ()  [unwired: 10 in, 1 out]
                n249 = call "Colour.vi"("result"="OK", "colourRef"=w350) -> ()  [unwired: 9 in, 1 out]
                n250 = call "设备状态.vi"("枚举"=enum16{"Read", "Write"}."Write", "Status_Write"=i16 80 ("设备状态")) -> ()  [unwired: 9 in, 1 out]
              }
              frame 81 {
                n251 = call "浮动通知.vi"("通知内容"="请放回检具8！" ("Status")) -> ()  [unwired: 11 in]
                n252 = call "设备状态.vi"("枚举"=enum16{"Read", "Write"}."Write", "Status_Write"=i16 83 ("设备状态")) -> ()  [unwired: 9 in, 1 out]
              }
              frame 85 {
                n253 = Index Array(array=w357, index=7 ("索引")) -> (element=w361:refnum<vi>)
                n254 = call "浮动通知.vi"("通知内容"="请拾取检具9！" ("Status")) -> ()  [unwired: 11 in]
                n255 = call "Colour.vi"("result"="OK", "colourRef"=w361) -> ()  [unwired: 9 in, 1 out]
                n256 = call "Colour.vi"("result"="等待") -> ()  [unwired: 10 in, 1 out]
                n257 = call "设备状态.vi"("枚举"=enum16{"Read", "Write"}."Write", "Status_Write"=i16 90 ("设备状态")) -> ()  [unwired: 9 in, 1 out]
              }
              frame 91 {
                n258 = call "浮动通知.vi"("通知内容"="请放回检具9！" ("Status")) -> ()  [unwired: 11 in]
                n259 = call "设备状态.vi"("枚举"=enum16{"Read", "Write"}."Write", "Status_Write"=i16 93 ("设备状态")) -> ()  [unwired: 9 in, 1 out]
              }
              frame 95 {
                n260 = Index Array(array=w368, index #1=8 ("索引")) -> (element #1=w373:refnum<vi>, element #2=w369:refnum<vi>)  [unwired: 1 in]
                n261 = call "浮动通知.vi"("通知内容"="请拾取检具10！" ("Status")) -> ()  [unwired: 11 in]
                n262 = call "Colour.vi"("result"="OK", "colourRef"=w373) -> ()  [unwired: 9 in, 1 out]
                n263 = call "Colour.vi"("result"="等待", "colourRef"=w369) -> ()  [unwired: 9 in, 1 out]
                n264 = call "设备状态.vi"("枚举"=enum16{"Read", "Write"}."Write", "Status_Write"=i16 100 ("设备状态")) -> ()  [unwired: 9 in, 1 out]
              }
              frame 101 {
                n265 = call "浮动通知.vi"("通知内容"="请放回检具10！" ("Status")) -> ()  [unwired: 11 in]
                n266 = call "设备状态.vi"("枚举"=enum16{"Read", "Write"}."Write", "Status_Write"=i16 103 ("设备状态")) -> ()  [unwired: 9 in, 1 out]
              }
              frame 105 {
                n267 = Index Array(array=w380, index #1=9 ("索引")) -> (element #1=w385:refnum<vi>, element #2=w381:refnum<vi>)  [unwired: 1 in]
                n268 = call "浮动通知.vi"("通知内容"="请拾取检具11！" ("Status")) -> ()  [unwired: 11 in]
                n269 = call "设备状态.vi"("枚举"=enum16{"Read", "Write"}."Write", "Status_Write"=i16 110 ("设备状态")) -> ()  [unwired: 9 in, 1 out]
                n270 = call "Colour.vi"("result"="OK", "colourRef"=w385) -> ()  [unwired: 9 in, 1 out]
                n271 = call "Colour.vi"("result"="等待", "colourRef"=w381) -> ()  [unwired: 9 in, 1 out]
              }
              frame 111 {
                n272 = call "浮动通知.vi"("通知内容"="请放回检具11！" ("Status")) -> ()  [unwired: 11 in]
                n273 = call "设备状态.vi"("枚举"=enum16{"Read", "Write"}."Write", "Status_Write"=i16 113 ("设备状态")) -> ()  [unwired: 9 in, 1 out]
              }
              frame 115 {
                n274 = Index Array(array=w392, index #1=10 ("索引")) -> (element #1=w397:refnum<vi>, element #2=w393:refnum<vi>)  [unwired: 1 in]
                n275 = call "浮动通知.vi"("通知内容"="请拾取检具12！" ("Status")) -> ()  [unwired: 11 in]
                n276 = call "Colour.vi"("result"="OK", "colourRef"=w397) -> ()  [unwired: 9 in, 1 out]
                n277 = call "Colour.vi"("result"="等待", "colourRef"=w393) -> ()  [unwired: 9 in, 1 out]
                n278 = call "设备状态.vi"("枚举"=enum16{"Read", "Write"}."Write", "Status_Write"=i16 120 ("设备状态")) -> ()  [unwired: 9 in, 1 out]
              }
              frame 121 {
                n279 = call "浮动通知.vi"("通知内容"="请放回检具12！" ("Status")) -> ()  [unwired: 11 in]
                n280 = call "设备状态.vi"("枚举"=enum16{"Read", "Write"}."Write", "Status_Write"=i16 123 ("设备状态")) -> ()  [unwired: 9 in, 1 out]
              }
              frame 125 {
                n281 = Index Array(array=w404, index #1=11 ("索引")) -> (element #1=w409:refnum<vi>, element #2=w405:refnum<vi>)  [unwired: 1 in]
                n282 = call "浮动通知.vi"("通知内容"="请拾取检具13！" ("Status")) -> ()  [unwired: 11 in]
                n283 = call "Colour.vi"("result"="OK", "colourRef"=w409) -> ()  [unwired: 9 in, 1 out]
                n284 = call "设备状态.vi"("枚举"=enum16{"Read", "Write"}."Write", "Status_Write"=i16 130 ("设备状态")) -> ()  [unwired: 9 in, 1 out]
                n285 = call "Colour.vi"("result"="等待", "colourRef"=w405) -> ()  [unwired: 9 in, 1 out]
              }
              frame 131 {
                n286 = call "浮动通知.vi"("通知内容"="请放回检具13！" ("Status")) -> ()  [unwired: 11 in]
                n287 = call "设备状态.vi"("枚举"=enum16{"Read", "Write"}."Write", "Status_Write"=i16 133 ("设备状态")) -> ()  [unwired: 9 in, 1 out]
              }
              frame 135 {
                n288 = Index Array(array=w416, index #1=12 ("索引")) -> (element #1=w421:refnum<vi>, element #2=w417:refnum<vi>)  [unwired: 1 in]
                n289 = call "浮动通知.vi"("通知内容"="请拾取检具14！" ("Status")) -> ()  [unwired: 11 in]
                n290 = call "Colour.vi"("result"="等待", "colourRef"=w417) -> ()  [unwired: 9 in, 1 out]
                n291 = call "Colour.vi"("result"="OK", "colourRef"=w421) -> ()  [unwired: 9 in, 1 out]
                n292 = call "设备状态.vi"("枚举"=enum16{"Read", "Write"}."Write", "Status_Write"=i16 140 ("设备状态")) -> ()  [unwired: 9 in, 1 out]
              }
              frame 141 {
                n293 = call "浮动通知.vi"("通知内容"="请放回检具14！" ("Status")) -> ()  [unwired: 11 in]
                n294 = call "设备状态.vi"("枚举"=enum16{"Read", "Write"}."Write", "Status_Write"=i16 143 ("设备状态")) -> ()  [unwired: 9 in, 1 out]
              }
              frame 145 {
                n295 = Index Array(array=w428, index #1=13 ("索引")) -> (element #1=w432:refnum<vi>, element #2=w429:refnum<vi>)  [unwired: 1 in]
                n296 = call "Colour.vi"("result"="等待", "colourRef"=w429) -> ()  [unwired: 9 in, 1 out]
                n297 = call "设备状态.vi"("枚举"=enum16{"Read", "Write"}."Write", "Status_Write"=i16 150 ("设备状态")) -> ()  [unwired: 9 in, 1 out]
                n298 = call "Colour.vi"("result"="OK", "colourRef"=w432) -> ()  [unwired: 9 in, 1 out]
              }
              frame 151 {
                n299 = call "设备状态.vi"("枚举"=enum16{"Read", "Write"}."Write", "Status_Write"=i16 153 ("设备状态")) -> ()  [unwired: 9 in, 1 out]
              }
              frame 155 {
                n300 = Index Array(array=w439, index=14 ("索引")) -> (element=w441:refnum<vi>)
                n301 = call "浮动通知.vi"("通知内容"="工艺完成！" ("Status")) -> ()  [unwired: 11 in]
                n302 = call "Colour.vi"("result"="OK", "colourRef"=w441) -> ()  [unwired: 9 in, 1 out]
                n303 = call "设备状态.vi"("枚举"=enum16{"Read", "Write"}."Write", "Status_Write"=i16 200 ("设备状态")) -> ()  [unwired: 9 in, 1 out]
              }
              frame 201 {
                n304 = global read "Global.vi" "检测结果"() -> (w450:refnum<vi>)
                n305 = global read "Global.vi" "结果显示字"() -> (w446:refnum<vi>)
                n306 = call "Colour.vi"("result"="NG", "colourRef"=w450) -> ()  [unwired: 9 in, 1 out]
                n307 = property class="Str"(reference=w446, "Value"="NG" ("值")) -> (reference out=w444:refnum<vi>)  [unwired: 1 in, 1 out]
                n308 = property class="Str"(reference=w444, "Text.TextColor"=u32 16711680) -> ()  [unwired: 1 in, 2 out]
                n309 = global read "Global1.vi" "联机模式"() -> (w449:enum16{"单机", "联网"})
                n310 = case shown="\"联网\"" w449 {
                  tunnel: ["报表" ("STEP") "录入数据库" ("STEP")] -> w448
                  frame "单机", Default {
                    n311 = call "设备状态.vi"("枚举"=enum16{"Read", "Write"}."Write", "Status_Write"=i16 6 ("设备状态")) -> ()  [unwired: 9 in, 1 out]
                  }
                  frame "联网" {
                  }
                }
                n312 = global write "Global1.vi" "生产结果"("NG" ("生产结果")) -> ()
                n313 = local write "STEP"(w448) -> ()
              }
              frame 202 {
                n314 = global read "Global.vi" "结果显示字"() -> (w459:refnum<vi>)
                n315 = global read "Global.vi" "检测结果"() -> (w463:refnum<vi>)
                n316 = property class="Str"(reference=w459, "Value"="OK" ("值")) -> (reference out=w457:refnum<vi>)  [unwired: 1 in, 1 out]
                n317 = call "Colour.vi"("result"="OK", "colourRef"=w463) -> ()  [unwired: 9 in, 1 out]
                n318 = property class="Str"(reference=w457, "Text.TextColor"=u32 6618880) -> ()  [unwired: 1 in, 2 out]
                n319 = global write "Global1.vi" "生产结果"("OK" ("生产结果")) -> ()
                n320 = global read "Global1.vi" "联机模式"() -> (w462:enum16{"单机", "联网"})
                n321 = case shown="\"单机\", 默认" w462 {
                  tunnel: ["报表" ("STEP") "录入数据库" ("STEP")] -> w460
                  frame "单机", Default {
                    n322 = call "设备状态.vi"("枚举"=enum16{"Read", "Write"}."Write", "Status_Write"=i16 6 ("设备状态")) -> ()  [unwired: 9 in, 1 out]
                  }
                  frame "联网" {
                  }
                }
                n323 = local write "STEP"(w460) -> ()
              }
              frame 1024 {
                n324 = call "浮动通知.vi"("通知内容"="急停！" ("Status")) -> ()  [unwired: 11 in]
                n325 = global read "Global.vi" "程序自动"() -> (w470:refnum<vi>)
                n326 = property class="Bool"(reference=w470, "Value"=FALSE) -> ()  [unwired: 1 in, 2 out]
              }
              frame 3721 {
                n327 = local write "STEP"("不合格锁定" ("STEP")) -> ()
                n328 = call "浮动通知.vi"("通知内容"="产品不合格程序锁定！" ("Status")) -> ()  [unwired: 11 in]
              }
              frame 3722 {
                n329 = global read "Global.vi" "程序自动"() -> (w475:refnum<vi>)
                n330 = call "浮动通知.vi"("通知内容"="授权成功，请复位！" ("Status")) -> ()  [unwired: 11 in]
                n331 = property class="Bool"(reference=w475, "Value"=FALSE) -> ()  [unwired: 1 in, 2 out]
              }
              frame 3723 {
                n332 = call "浮动通知.vi"("通知内容"="请取出不合格产品并摆放至不合格品区！" ("Status")) -> ()  [unwired: 11 in]
              }
            }
          }
          frame "不合格锁定" {
            n333 = call "临时授权.vi"() -> ("授权成功"=w479:bool)  [unwired: 11 in]
            n334 = case shown="假" w479 {
              frame False {
              }
              frame True {
                n335 = local write "STEP"("报表" ("STEP")) -> ()
                n336 = call "设备状态.vi"("枚举"=enum16{"Read", "Write"}."Write", "Status_Write"=i16 3722 ("设备状态")) -> ()  [unwired: 9 in, 1 out]
              }
            }
            n337 = Wait (ms)(milliseconds to wait=u32 100 ("等待时间（毫秒）")) -> ()  [unwired: 1 out]
          }
          frame "报表" {
            n338 = global read "Global1.vi" "生产结果"() -> (w488:string)
            n339 = global read "Global1.vi" "工位追溯码"() -> (w485:string)
            n340 = call "Report.vi"("文件重命名"=TRUE, "文件名称"=w485) -> ()  [unwired: 9 in, 1 out]
            n341 = case shown="\"OK\"" w488 {
              frame "NG", Default {
              }
              frame "OK" {
                n342 = global read "Global.vi" "合格数量"() -> (w495:refnum<vi>)
                n343 = property class="Num"(reference=w495) -> (reference out=w494:refnum<vi>, error out=w493:errorcluster, "Value"=w492:variant)  [unwired: 1 in]
                n344 = Variant To Data(type=u32 0, Variant=w492) -> (data=w491:u32)  [unwired: 1 in, 1 out]
                n345 = Increment(x=w491) -> (x+1=w490:u32)
                n346 = property class="Num"(reference=w494, error in=w493, "Value"=w490) -> ()  [unwired: 2 out]
              }
            }
            n347 = call "设备状态.vi"("枚举"=enum16{"Read", "Write"}."Write", "Status_Write"=i16 6 ("设备状态")) -> ()  [unwired: 9 in, 1 out]
            n348 = local write "STEP"("自动" ("STEP")) -> ()
          }
        }
        n349 = Wait Until Next ms Multiple(millisecond multiple=u32 10 ("毫秒倍数")) -> ()  [unwired: 1 out]
        n350 = global read "Global.vi" "程序关闭"() -> (w33:bool)
      }
      n351 = while {
        stop <- w496 stop-if-true
        n352 = event shown="[1] 前面板关闭" {
          selector: _ -> [_ _]
          dyn-events: _ -> [_ _]
          timeout: 100 -> [_ _]
          event Timeout {
            n353 = event-data() -> ()  [unwired: 1 in, 3 out]
            n354 = stacked-sequence {
              frame #0 {
                n355 = shared-variable "我的电脑\\A17031611.lvlib\\错误代码"() -> (w498:u16)  [unwired: 1 in, 1 out]
                n356 = feedback #1() -> (w508:u16)  [unwired: 1 in]
                n357 = feedback-in #1(w498) -> ()
                n358 = case shown="0" w498 {
                  frame 0 {
                    n359 = global read "Global.vi" "报警图标"() -> (w509:refnum<vi>)
                    n360 = property class="Bool"(reference=w509, "Visible"=FALSE ("可见")) -> ()  [unwired: 1 in, 2 out]
                  }
                  frame 1, Default {
                    n361 = global read "Global.vi" "报警图标"() -> (w512:refnum<vi>)
                    n362 = property class="Bool"(reference=w512, "Visible"=TRUE ("可见")) -> ()  [unwired: 1 in, 2 out]
                  }
                }
                n363 = Greater Or Equal?(x=w498, y=i16 5000) -> (x >= y?=w506:bool)
                n364 = Less?(x=w498, y=i16 5200) -> (x < y?=w507:bool)
                n365 = Equal?(x=w498, y=w508) -> (x = y?=w505:bool)
                n366 = global read "Global.vi" "报警图标"() -> (w500:refnum<vi>)
                n367 = And(x=w506, y=w507) -> (x .and. y?=w499:bool)
                n368 = property class="Bool"(reference=w500, "Value"=w499) -> ()  [unwired: 1 in, 2 out]
                n369 = Bundle By Name(cluster=errorcluster {"status"=FALSE, "code"=0, "source"=""} ("错误常量"), "status"=w499, "code"=w498) -> (w504:errorcluster)
                n370 = case shown="真" w505 {
                  tunnel: w504 -> [w513 _]
                  frame False {
                    n371 = call "报警处理.vi"("错误常量"=w513) -> ()  [unwired: 9 in, 2 out]
                  }
                  frame True {
                  }
                }
              }
              frame #1 {
                n372 = disable-structure shown="禁用" {
                  frame Disabled {
                    n373 = global read "Global.vi" "程序自动"() -> (w517:refnum<vi>)
                    n374 = property class="Bool"(reference=w517) -> ("Value"=w516:variant)  [unwired: 1 in, 2 out]
                    n375 = Variant To Data(type=FALSE, Variant=w516) -> (data=w514:bool)  [unwired: 1 in, 1 out]
                    n376 = case shown="真" w514 {
                      selector: w514 -> [w519 _]
                      frame False {
                        n377 = call <userlib>:"Boolean Trigger__ogtk.vi"("Boolean Input"=w519) -> ("Rising Edge"=w518:bool)  [unwired: 1 in, 1 out]
                        n378 = case shown="真" w518 {
                          frame False {
                          }
                          frame True {
                            n379 = local write "STEP"("手动" ("STEP")) -> ()
                          }
                        }
                      }
                      frame True {
                        n380 = shared-variable "我的电脑\\A17031611.lvlib\\设备状态"() -> (w521:i16)  [unwired: 1 in, 1 out]
                        n381 = case shown="5" w521 {
                          frame 0, Default {
                            n382 = global read "Global.vi" "程序自动"() -> (w523:refnum<vi>)
                            n383 = call "浮动通知.vi"("通知内容"="请复位") -> ()  [unwired: 11 in]
                            n384 = property class="Bool"(reference=w523, "Value"=FALSE) -> ()  [unwired: 1 in, 2 out]
                          }
                          frame 5 {
                            n385 = local write "STEP"("初始化" ("STEP")) -> ()
                          }
                        }
                      }
                    }
                  }
                  frame Enabled {
                  }
                }
              }
            }
          }
          event Panel Close {
            n386 = event-data() -> ()  [unwired: 1 in, 4 out]
            n387 = global write "Global.vi" "程序关闭"(TRUE ("程序关闭")) -> ()
          }
        }
        n388 = global read "Global.vi" "程序关闭"() -> (w496:bool)
      }
    }
  }
